vi "Gasflasche Cluster in Text.vi"(10 "Gasflasche":T2={"Gasflasche"={"Gasname für die Auswahl"="", "Chargennummer"="", "Ablaufdatum"=timestamp(0 s since 1904-01-01)}, "Trägergas"="N2", "Komponenten"=[]} {"Gasflasche"."Ablaufdatum" format="%<%d.%m.%Y>T"; "Komponenten"."Konzentration IST" format="%#.4f"; "Komponenten"."Genauigkeit" format="%#.1f"}) -> (2 "Gasflasche Text Array":T1[](array[typedef]))   [LabVIEW 2020, in "System Einstellungen V2.lvlib"]
uses:
  System Einstellungen V2.lvlib
  Gasflasche gesamt.ctl
  Gasflasche.ctl
  Traegergas.ctl
  Gasflaschenkomponente.ctl
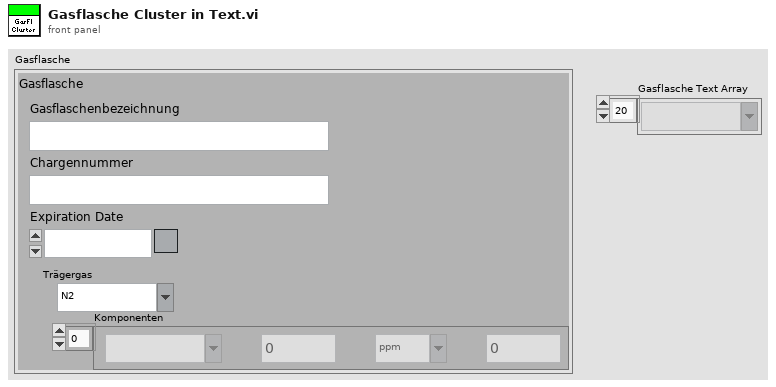
[diagram p1: front panel]
types:
  T1 = typedef "System Einstellungen V2.lvlib/Traegergas.ctl" = string
  T2 = typedef "System Einstellungen V2.lvlib/Gasflasche gesamt.ctl" = cluster{"Gasflasche":T3, "Trägergas":T1, "Komponenten":T4[]}
  T3 = typedef "System Einstellungen V2.lvlib/Gasflasche.ctl" = cluster{"Gasname für die Auswahl":string, "Chargennummer":string, "Ablaufdatum":timestamp}
  T4 = typedef "System Einstellungen V2.lvlib/Gasflaschenkomponente.ctl" = cluster{"Gasauswahl":string, "Konzentration IST":dbl, "Einheit":string, "Genauigkeit":dbl}
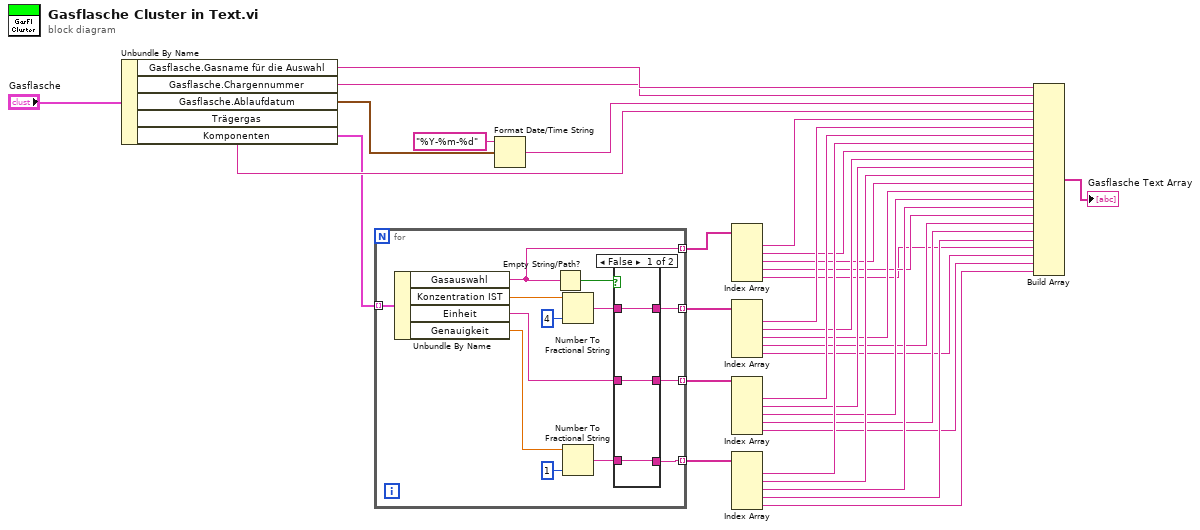
[diagram p0: block diagram]
diagram:
  n1 = Unbundle By Name("Gasflasche") -> ("Gasflasche.Gasname für die Auswahl"=w31:string, "Gasflasche.Chargennummer"=w30:string, "Gasflasche.Ablaufdatum"=w29:timestamp, "Trägergas"=w27:T1, "Komponenten"=w25:T4[])
  n2 = for {
    tunnel: w25 -> [w45] mode=indexing
    tunnel: [w41] -> w24 mode=indexing
    tunnel: [w39] -> w22 mode=indexing
    tunnel: [w34] -> w18 mode=indexing
    tunnel: [w36] -> w20 mode=indexing
    n3 = Unbundle By Name(w45) -> ("Gasauswahl"=w41:string, "Konzentration IST"=w44:dbl, "Einheit"=w37:string, "Genauigkeit"=w42:dbl)
    n4 = Empty String/Path?(string/path=w41) -> (empty?=w40:bool)
    n5 = Number To Fractional String(number=w44, precision (6)=i16 4 ("Genauigkeit (6)")) -> (F-format string=w38:string)  [unwired: 2 in]
    n6 = Number To Fractional String(number=w42, precision (6)=i16 1 ("Genauigkeit (6)")) -> (F-format string=w35:string)  [unwired: 2 in]
    n7 = case shown="False" w40 {
      tunnel: [w49 _] -> w39
      tunnel: w38 -> [w49 _]
      tunnel: w37 -> [w48 _]
      tunnel: [w48 _] -> w36
      tunnel: w35 -> [w47 _]
      tunnel: [w47 _] -> w34
      frame False {
      }
      frame True {
      }
    }
  }
  n8 = Format Date/Time String(time format string (%c)="%Y-%m-%d" ("Zeitformatierungs-String (%c)"), seconds (now)=w29) -> (date/time string=w28:string)  [unwired: 1 in]
  n9 = Index Array(array=w24) -> (element #1=w23:string, element #2=w16:string, element #3=w12:string, element #4=w8:string, element #5=w4:string)  [unwired: 5 in]
  n10 = Index Array(array=w22) -> (element #1=w21:string, element #2=w15:string, element #3=w11:string, element #4=w7:string, element #5=w3:string)  [unwired: 5 in]
  n11 = Index Array(array=w20) -> (element #1=w19:string, element #2=w14:string, element #3=w10:string, element #4=w6:string, element #5=w2:string)  [unwired: 5 in]
  n12 = Index Array(array=w18) -> (element #1=w17:string, element #2=w13:string, element #3=w9:string, element #4=w5:string, element #5=w1:string)  [unwired: 5 in]
  n13 = Build Array(w31, w30, w28, w27, w23, w21, w19, w17, w16, w15, w14, w13, w12, w11, w10, w9, w8, w7, w6, w5, w4, w3, w2, w1) -> (→"Gasflasche Text Array":T1[])
